vi "Check Init SSE Handler.vi"(8 "error in (no error)":errorcluster, 11 "Server in":refnum<class "Server.lvclass">) -> (0 "error out":errorcluster, 3 "Server out":refnum<class "Server.lvclass">)   [LabVIEW 2020, in "HTTP Server.lvlib" / "Server.lvclass"]
uses:
  Server.lvclass
  Server.lvclass/Server.ctl
  SSE Handler/SSE Handler.lvclass
  C:/dev/lv20CE/relink/lv-http-server/HTTP Server/Handler/Handler.lvclass
  Add Connection Handler.vi
  Add Request Handler.vi
  Add Route Handler.vi
  Add Controller Handler.vi
  Add Controller.vi
  Add Response Handler.vi
  Add Complete Handler.vi
  Add Exception Handler.vi
  Connection Handler/Connection Handler.lvclass
  Request Handler/Request Handler.lvclass
  Route Handler/Route Handler.lvclass
  Controller Handler/Controller Handler.lvclass
  Controller/Controller.lvclass
  Response Handler/Response Handler.lvclass
  Complete Handler/Complete Handler.lvclass
  Exception Handler/Exception Handler.lvclass
  Handler/Handler.lvclass
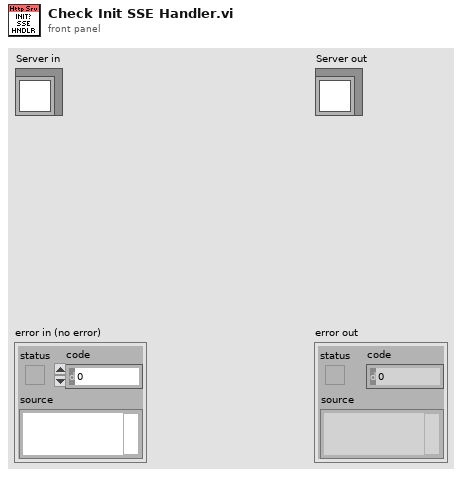
[diagram p1: front panel]
types:
  T1 = typedef "HTTP Server.lvlib/Server.lvclass/Ref Data.ctl" = cluster{"Connection Handler Map":T2, "Request Handler Map":T4, "Route Handler Map":T5, "Controller Handler Map":T6, "Controller Map":T7, "Response Handler Map":T8, "Complete Handler Map":T9, "Exception Handler Map":T10, "Connection Handler Index":u16, "Request Handler Index":u16, "Route Handler Index":u16, "Controller Handler Index":u16, "Controller Index":u16, "Response Handler Index":u16, "Complete Handler Index":u16, "Exception Handler Index":u16, "Values":refnum<class "Values.lvclass">, "Path":path, "Session Type":refnum<class "Session.lvclass">, "Session Cookie Name":string, "WebSocket Handler":refnum<class "WebSocket Handler.lvclass">, "WebSocket Handling":bool, "SSE Handler":refnum<class "SSE Handler.lvclass">, "SSE Handling":bool}
  T2 = typedef "HTTP Server.lvlib/Connection Handler Map.ctl" = map{T3, refnum<class "Connection Handler.lvclass">}
  T3 = typedef "HTTP Server.lvlib/Priority.ctl" = cluster{"Entity":u16, "Index":u16}
  T4 = typedef "HTTP Server.lvlib/Request Handler Map.ctl" = map{T3, refnum<class "Request Handler.lvclass">}
  T5 = typedef "HTTP Server.lvlib/Route Handler Map.ctl" = map{T3, refnum<class "Route Handler.lvclass">}
  T6 = typedef "HTTP Server.lvlib/Controller Handler Map.ctl" = map{T3, refnum<class "Controller Handler.lvclass">}
  T7 = typedef "HTTP Server.lvlib/Controller Map.ctl" = map{T3, refnum<class "Controller.lvclass">}
  T8 = typedef "HTTP Server.lvlib/Response Handler Map.ctl" = map{T3, refnum<class "Response Handler.lvclass">}
  T9 = typedef "HTTP Server.lvlib/Complete Handler Map.ctl" = map{T3, refnum<class "Complete Handler.lvclass">}
  T10 = typedef "HTTP Server.lvlib/Exception Handler Map.ctl" = map{T3, refnum<class "Exception Handler.lvclass">}
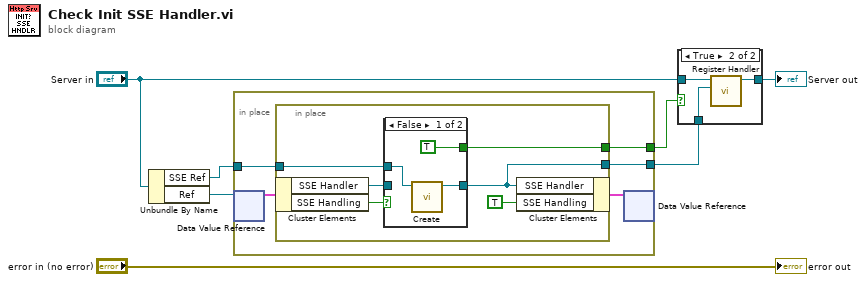
[diagram p0: block diagram]
diagram:
  n1 = Unbundle By Name("Server in") -> ("SSE Ref"=w5:refnum<data-value>, "Ref"=w6:refnum<data-value>)
  n2 = in-place {
    in-place-border: w5 -> [w10]
    in-place-border: [w9] -> w2
    in-place-border: [w8] -> w1
    n3 = in-place-dvr #1(w6) -> (w12:T1)  [unwired: 1 out]
    n4 = in-place {
      in-place-border: w10 -> [w15]
      in-place-border: [w14] -> w9
      in-place-border: [w13] -> w8
      n5 = in-place-cluster #2(w12) -> ("SSE Handler"=w18:refnum<class "SSE Handler.lvclass">, "SSE Handling"=w17:bool)
      n6 = case shown="False" w17 {
        tunnel: w18 -> [_ w22]
        tunnel: [w21 w22] -> w14
        tunnel: w15 -> [w20 _]
        tunnel: [TRUE _] -> w13
        frame False {
          n7 = call "Create.vi"("SSE Ref"=w20) -> ("SSE Handler out"=w21:refnum<class "SSE Handler.lvclass">)  [unwired: 9 in, 1 out]
        }
        frame True {
        }
      }
      n8 = in-place-cluster #2("SSE Handler"=w14, "SSE Handling"=TRUE ("WebSocket Handling")) -> (w11:T1)
    }
    n9 = in-place-dvr #1(w11) -> ()  [unwired: 2 out]
  }
  n10 = case shown="True" w1 {
    tunnel: "Server in" -> [w23 w26]
    tunnel: [w23 w25] -> w3
    tunnel: w2 -> [_ w24]
    frame False {
    }
    frame True {
      n11 = call "Register Handler.vi"("Handler"=w24, "Server in"=w26) -> ("Server out"=w25:refnum<class "Server.lvclass">)  [unwired: 8 in, 1 out]
    }
  }
  "Server out" <- w3
  "error out" <- "error in (no error)"
